vi "GetStatus.vi"(8 "error in (no error)":errorcluster, 11 "Instrument.VRM in":refnum<class "Instrument.OxfordVRM.lvclass">) -> (0 "error out":errorcluster, 1 "Status (ALL)":T1, 2 "Status":string[](array[string]), 3 "Instrument.VRM out":refnum<class "Instrument.OxfordVRM.lvclass">)   [LabVIEW 2019, in "Instrument.OxfordVRM.lvclass"]
doc: "Status Bits:\n[0] = Hold?\n[1] = Ramp to Set?\n[2] = Ramp to Zero?\n[3] = Clamp?"
uses:
  Instrument.OxfordVRM.lvclass
  Typedefs/Instrument.VRM.protectedCommands-enum.ctl
  ef272791-987c-496b-baec-840fbed0f584.vi
  Typedefs/Instrument.VRM.GetStatus--cluster.ctl
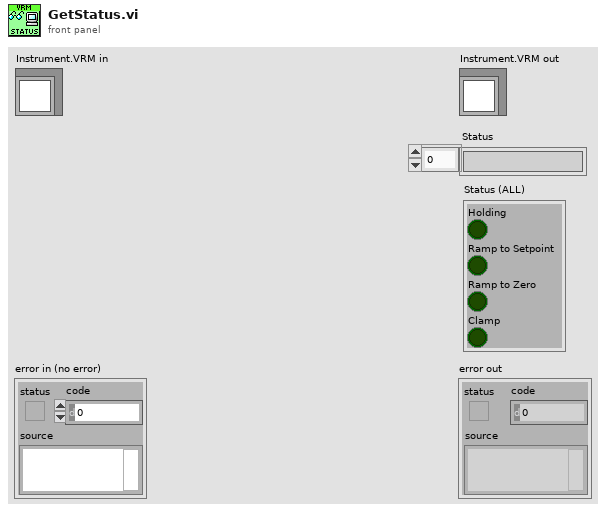
[diagram p1: front panel]
types:
  T1 = cluster{"Holding":bool, "Ramp to Setpoint":bool, "Ramp to Zero":bool, "Clamp":bool}
  T2 = typedef "Instrument.OxfordVRM.lvclass/Instrument.VRM.GetStatus--cluster.ctl" = cluster{"Status":string[]}
  T3 = typedef "Instrument.OxfordVRM.lvclass/Instrument.VRM.protectedCommands-enum.ctl" = enum16{"Hold", "RampToSet", "RampToZero", "Clamp", "SetTarget", "GetStatus", "GetTarget", "GetField"}
  T4 = cluster{"[0]":bool, "[1]":bool, "[2]":bool, "[3]":bool}
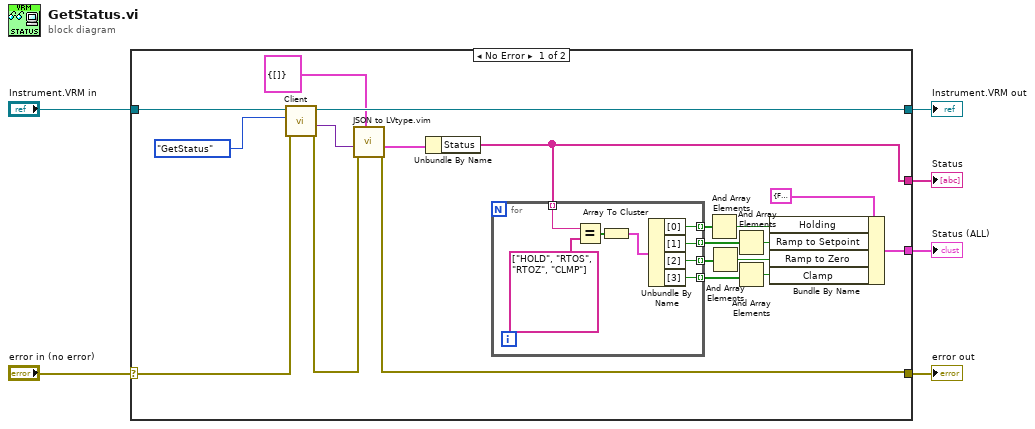
[diagram p0: block diagram]
diagram:
  n1 = case shown="No Error" "error in (no error)" {
    selector: "error in (no error)" -> [w14 w36]
    tunnel: [w9 w36] -> w5
    tunnel: [w12 w35] -> w3
    tunnel: "Instrument.VRM in" -> [w15 w35]
    tunnel: [w7 _] -> w2
    tunnel: [w17 _] -> w1
    frame No Error {
      n2 = call-dynamic "Client.vi"("error in (no error)"=w14, "Command in"=Instrument.VRM.protectedCommands-enum."GetStatus" ("protectedCommands"), "Instrument in"=w15) -> ("error out"=w10:errorcluster, "Data out"=w16:variant, "Instrument out"=w12:refnum<class "Instrument.OxfordVRM.lvclass">)  [unwired: 5 in, 1 out]
      n3 = call "JSON to LVtype.vim"("type"=T2 {"Status"=[]} ("GetStatus"), "error in (no error)"=w10, "JSON Data in"=w16) -> ("error out"=w9:errorcluster, "Data out"=w11:T2)  [unwired: 7 in]
      n4 = Unbundle By Name(w11) -> ("Status"=w7:string[])
      n5 = for {
        tunnel: w7 -> [w32] mode=indexing
        tunnel: [w30] -> w26 mode=indexing
        tunnel: [w29] -> w25 mode=indexing
        tunnel: [w28] -> w24 mode=indexing
        tunnel: [w27] -> w23 mode=indexing
        n6 = Equal?(x=w32, y=string[] ["HOLD", "RTOS", "RTOZ", "CLMP"] ("Array")) -> (x = y?=w34:bool[])
        n7 = Array To Cluster(array=w34) -> (cluster=w31:T4)
        n8 = Unbundle By Name(w31) -> ("[0]"=w30:bool, "[1]"=w29:bool, "[2]"=w28:bool, "[3]"=w27:bool)
      }
      n9 = And Array Elements(Boolean array=w26) -> (logical AND=w18:bool)
      n10 = And Array Elements(Boolean array=w24) -> (logical AND=w20:bool)
      n11 = And Array Elements(Boolean array=w25) -> (logical AND=w19:bool)
      n12 = And Array Elements(Boolean array=w23) -> (logical AND=w21:bool)
      n13 = Bundle By Name(cluster=T1 {"Holding"=FALSE, "Ramp to Setpoint"=FALSE, "Ramp to Zero"=FALSE, "Clamp"=FALSE} ("Status"), "Holding"=w18, "Ramp to Setpoint"=w19, "Ramp to Zero"=w20, "Clamp"=w21) -> (w17:T1)
    }
    frame Error {
    }
  }
  "error out" <- w5
  "Instrument.VRM out" <- w3
  "Status" <- w2
  "Status (ALL)" <- w1
